vi "Example Simple.vi"() -> ()   [LabVIEW 2010]
uses:
  C:/tf/play/labview/Tinkerforge.dll
panel:
  in  "uid":string="ctG"
  in  "port":i32=4223
  in  "host":string="localhost"
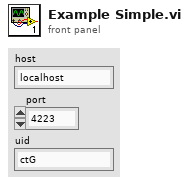
[diagram p1: front panel]
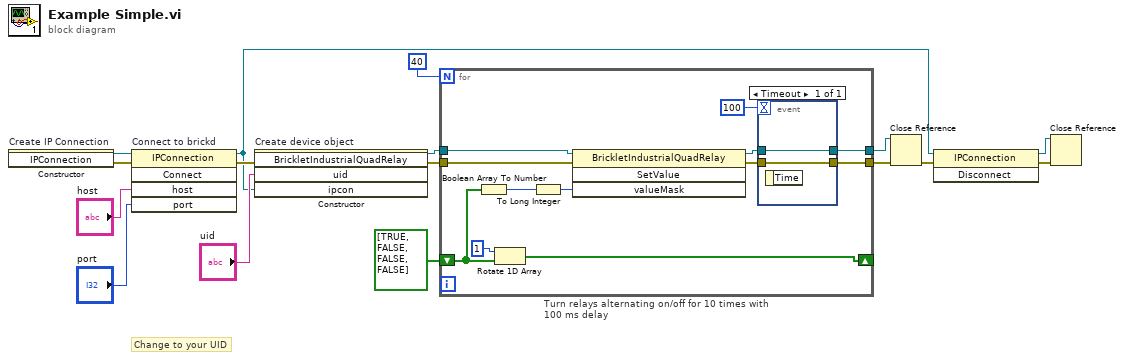
[diagram p0: block diagram]
diagram:
  # "Change to your UID"
  n1 = constructor on="Create IP Connection" class="IPConnection"() -> (reference out=w16:refnum<k24>, error out=w7:errorcluster)  [unwired: 3 in, 1 out]
  n2 = invoke on="Connect to brickd" class="IPConnection" method="Connect"(reference=w16, error in=w7, "host"="host", "port"="port") -> (reference out=w9:refnum<k24>, error out=w12:errorcluster)  [unwired: 1 in, 3 out]
  n3 = constructor on="Create device object" class="BrickletIndustrialQuadRelay"(error in=w12, "uid"="uid", "ipcon"=w9) -> (reference out=w4:refnum<k24>, error out=w5:errorcluster)  [unwired: 2 in, 3 out]
  n4 = for "Turn relays alternating on/off for 10 times with 100 ms delay" {
    N: 40 -> [_]
    tunnel: w5 -> [w28]
    tunnel: w4 -> [w27]
    tunnel: [w23] -> w3
    tunnel: [w25] -> w2
    shift-right: [w17] -> _
    shift-left: bool[] [TRUE, FALSE, FALSE, FALSE] -> [w18]
    n5 = Boolean Array To Number(Boolean array=w18) -> (number=w21:u32)
    n6 = Rotate 1D Array(1:w18, 2:1 ("n")) -> (0:w17:bool[])
    n7 = To Long Integer(number=w21) -> (32bit integer=w20:i32)
    n8 = invoke class="BrickletIndustrialQuadRelay" method="SetValue"(reference=w27, error in=w28, "valueMask"=w20) -> (reference out=w24:refnum<k24>, error out=w22:errorcluster)  [unwired: 1 in, 2 out]
    n9 = event shown="[0] Timeout" {
      selector: _ -> [_]
      dyn-events: _ -> [_]
      timeout: 100 -> [_]
      tunnel: [w30] -> w25
      tunnel: w24 -> [w30]
      tunnel: [w29] -> w23
      tunnel: w22 -> [w29]
      event Timeout {
        n10 = event-data() -> ()  [unwired: 1 in, 1 out]
      }
    }
  }
  n11 = Close Reference(reference=w2, error in (no error)=w3) -> (error out=w11:errorcluster)
  n12 = invoke class="IPConnection" method="Disconnect"(reference=w9, error in=w11) -> (reference out=w8:refnum<k24>, error out=w10:errorcluster)  [unwired: 1 in, 1 out]
  n13 = Close Reference(reference=w8, error in (no error)=w10) -> ()  [unwired: 1 out]
